vi "Calculate PulseEn Parameters.vi"(10 "PAEN Timing In":T1={"tRF (s)"=0.0, "Duty Cycle"=50.0, "t1 (s)"=5e-07, "t2 (s)"=5e-07, "t3 (s)"=0.0, "Period (s)"=0.0, "WLAN PFI Mode"=enum."Static"} {"Period (s)" format="%#_5p"; "t3 (s)" min=0.0 step=0.01 format="%#_5p"; "t2 (s)" min=0.0 max=0.1 step=0.01 format="%#_3p"; "t1 (s)" min=0.0 max=0.1 step=0.01 format="%#_3p"; "Duty Cycle" min=1.0 max=100.0 step=1.0 format="%#_2d%%"; "tRF (s)" min=0.0 step=0.01 format="%#_5p"}) -> (2 "PAEN Timing Out":T1={"tRF (s)"=0.0, "Duty Cycle"=50.0, "t1 (s)"=5e-07, "t2 (s)"=5e-07, "t3 (s)"=0.0, "Period (s)"=0.0, "WLAN PFI Mode"=enum."Static"} {"Period (s)" format="%#_5p"; "t3 (s)" min=0.0 step=0.01 format="%#_5p"; "t2 (s)" min=0.0 max=0.1 step=0.01 format="%#_3p"; "t1 (s)" min=0.0 max=0.1 step=0.01 format="%#_3p"; "Duty Cycle" min=1.0 max=100.0 step=1.0 format="%#_2d%%"; "tRF (s)" min=0.0 step=0.01 format="%#_5p"})   [LabVIEW 2018, in "RDLUtilities.lvlib"]
uses:
  RDLUtilities.lvlib
  SG/Typedefs/PAEN Timing.ctl
  SG/SG.lvlib
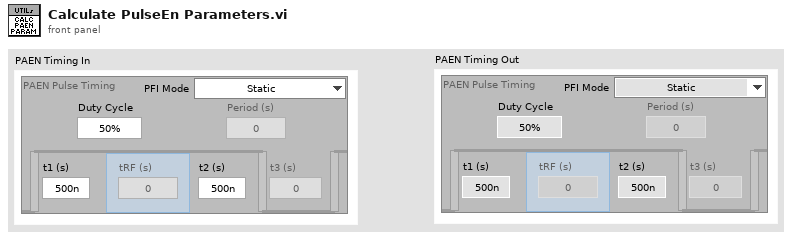
[diagram p1: front panel]
types:
  T1 = typedef "SG.lvlib/PAEN Timing.ctl" = cluster{"tRF (s)":dbl, "Duty Cycle":dbl, "t1 (s)":dbl, "t2 (s)":dbl, "t3 (s)":dbl, "Period (s)":dbl, "WLAN PFI Mode":enum16{"Static", "Dynamic"}}
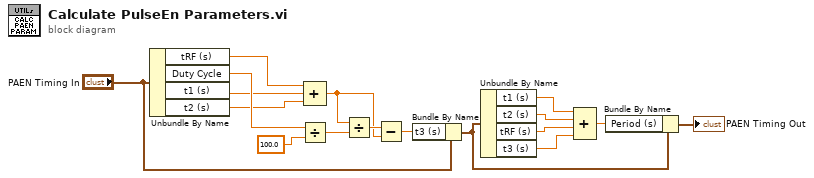
[diagram p0: block diagram]
diagram:
  n1 = Unbundle By Name("PAEN Timing In") -> ("tRF (s)"=w7:dbl, "Duty Cycle"=w6:dbl, "t1 (s)"=w5:dbl, "t2 (s)"=w4:dbl)
  n2 = Divide(x=w6, y=100.0) -> (x/y=w16:dbl)
  n3 = Compound Arithmetic op=ADD(w7, w5, w4) -> (w13:dbl)
  n4 = Divide(x=w13, y=w16) -> (x/y=w14:dbl)
  n5 = Subtract(x=w14, y=w13) -> (x-y=w12:dbl)
  n6 = Bundle By Name(cluster="PAEN Timing In", "t3 (s)"=w12) -> (w17:T1)
  n7 = Unbundle By Name(w17) -> ("t1 (s)"=w11:dbl, "t2 (s)"=w10:dbl, "tRF (s)"=w9:dbl, "t3 (s)"=w8:dbl)
  n8 = Compound Arithmetic op=ADD(w11, w10, w9, w8) -> (w3:dbl)
  n9 = Bundle By Name(cluster=w17, "Period (s)"=w3) -> (→"PAEN Timing Out":T1)
